vi "Volume Mul.vi"(8 "error in (no error)":errorcluster, 11 "RGetInputVolume in":refnum<class "RGetInputVolume.lvclass">) -> (0 "error out":errorcluster, 2 "Volume Mul":dbl, 3 "RGetInputVolume out":refnum<class "RGetInputVolume.lvclass">)   [LabVIEW 2020, in "obs-websocket.lvlib" / "RGetInputVolume.lvclass"]
uses:
  RGetInputVolume.lvclass
  RGetInputVolume.lvclass/RGetInputVolume.ctl
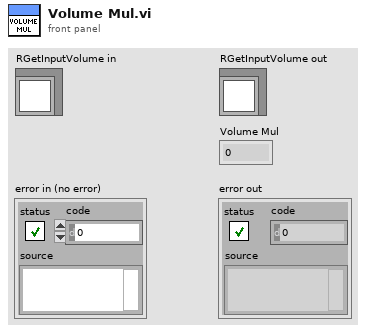
[diagram p1: front panel]
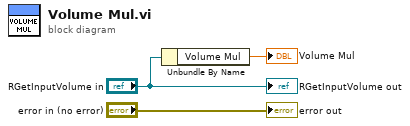
[diagram p0: block diagram]
diagram:
  n1 = Unbundle By Name("RGetInputVolume in") -> ("Volume Mul"=→"Volume Mul":dbl)
  "error out" <- "error in (no error)"
  "RGetInputVolume out" <- "RGetInputVolume in"
